vi "ATR.vi"() -> ()   [LabVIEW 2017]
panel:
  out "ATR 2":string[][](table)=[["Test Communication", "-", "-", "-", "-", ""], ["Set S/N", "-", "-", "-", "-", ""], ["Set Board Number", "-", "-", "-", "-", ""], [" ", "", "", "", "", ""], ["Test Communication", "-", "-", "-", "-", ""], ["Get S/N", "-", "-", "-", "", ""], ["Get Board Number", "-", "-", "-", "", ""], ["Get FW", "-", "-", "-", "", ""], ["Enable Motor", "", "", "", "", ""], ["Small position command", "", "", "", "", ""], ["Measure delta", "", "", "", "", ""], ["Velocity command", "", "", "", "", ""]] caption="ATR"
  out "ATR":string[][](table)=[["Test Communication", "-", "-", "-", "-", ""], ["Set S/N", "-", "-", "-", "-", ""], ["Set Board Number", "-", "-", "-", "-", ""], [" ", "", "", "", "", ""], ["Test Communication", "-", "-", "-", "-", ""], ["Get S/N", "-", "-", "-", "", ""], ["Get Board Number", "-", "-", "-", "", ""], ["Get FW", "-", "-", "-", "", ""], ["Enable Motor", "", "", "", "", ""], ["Small position command", "", "", "", "", ""], ["Measure delta", "", "", "", "", ""], ["Velocity command", "", "", "", "", ""]]
  out "Array 2":string[](array[string])
  out "Array":string[](array[string])
  out "deleted portion 2":string[](array[string])
  out "deleted portion":string[](array[string])
  out "ArrAHU":string[][](array[string])
  out "ArrEbay":string[][](array[string])
  out "Mort Temp":string[][](array[string])
  out "Aux":string[][](array[string])
  out "Burnin":string[][](array[string])
  out "Temp Algo":string[][](array[string])
  out "Speed":string[][](array[string])
  out "Tempreature calibration":string[][](array[string])
  out "StopTime":string[][](array[string])
  out "Enable":string[][](array[string])
  out "Communication":string[][](array[string])
  out "Visual Inspection":string[][](array[string])
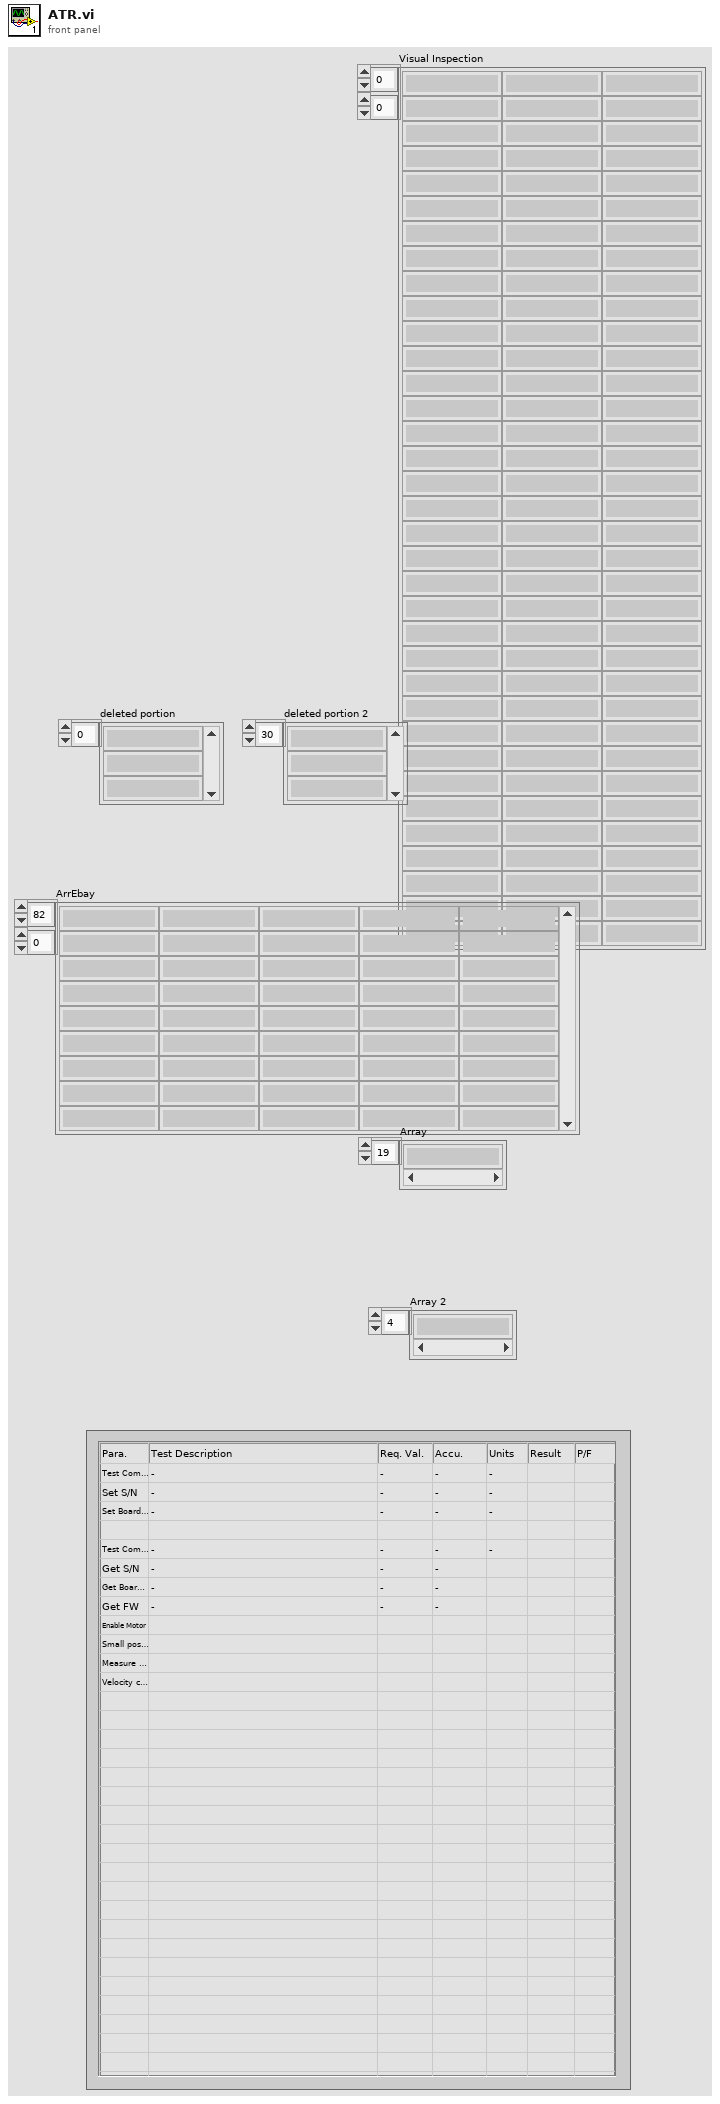
[diagram p1: front panel]
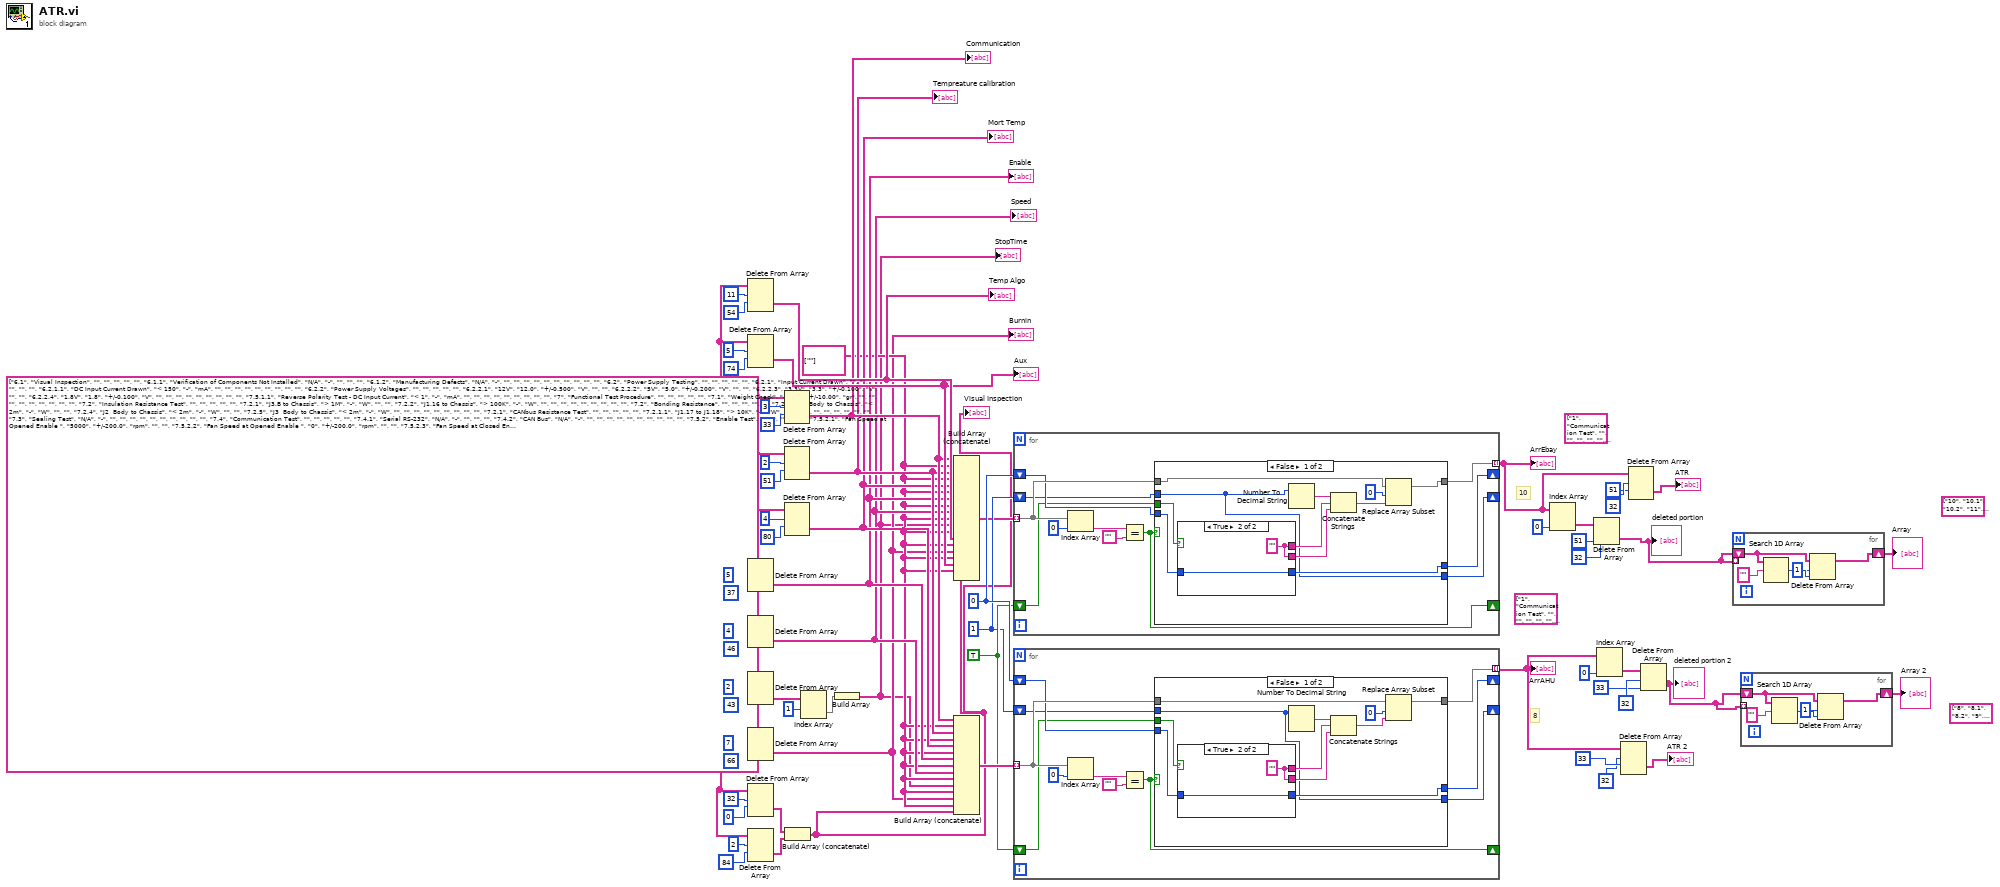
[diagram p0: block diagram]
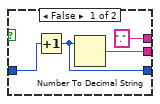
[diagram p2: hidden frame]
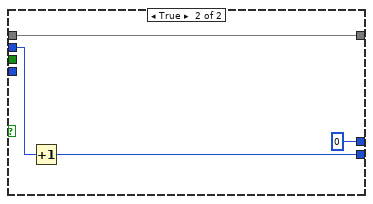
[diagram p3: hidden frame]
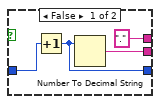
[diagram p4: hidden frame]
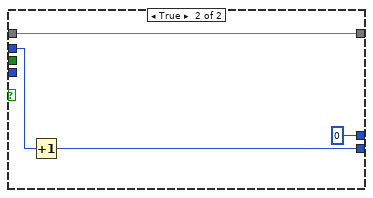
[diagram p5: hidden frame]
diagram:
  (unwired) string[] ["8", "8.1", "8.2", "9", "9.1", "9.2", "10", "10.1", "10.2", "10.3", "10.4", "11", "12", "12.1", "13", "13.1", "13.2", "14", "14.1", "14.2", "14.3", "15", "15.1", "16"] ("Array 3")
  (unwired) string[] ["10", "10.1", "10.2", "11", "11.1", "11.2", "12", "12.1", "12.2", "12.3", "12.4", "13", "14", "14.1", "15", "15.1", "15.2", "16", "16.1", "16.2", "16.3", "17", "17.1", "18"] ("Array 4")
  (unwired) string[][] [["1", "Communication Test", "", "", "", "", ""], ["1.1", "Serial RS-232", "N/A", "-", "", "", ""], ["1.2", "CAN Bus", "N/A", "-", "", "", ""], ["", "", "", "", "", "", ""], ["2", "Temperature Sensor Calibration", "", "", "", "", ""], ["2.1", "Sensor Reading Analog Offset", "0", "+/-0.100", ".", "", ""], ["", "", "", "", "", "", ""], ["3", "Motor Termistor Input Test", "", "", "", "", ""], ["3.1", "60 Degree", "60", "+/-3.00", "C", "", ""], ["3.2", "90 Degree", "90", "+/-3.00", "C", "", ""], ["3.3", "120 Degree", "120", "+/-3.00", "C", "", ""], ["", "", "", "", "", "", ""], ["4", "Enable Test", "", "", "", "", ""], ["4.1", "Fan Speed at Opened Enable ", "5000", "+/-200.0", "rpm", "", ""], ["4.2", "Fan Speed at Opened Enable ", "0", "+/-200.0", "rpm", "", ""], ["4.3", "Fan Speed at Closed Enable ", "5000", "+/-200.0", "rpm", "", ""], ["4.4", "Motor Rotation Direction", "Counter-clockwise (Inlet)", "-", "", "", ""], ["", "", "", "", "", "", ""], ["5", "Speed Command Test", "", "", "", "", ""], ["5.1", "Fan Speed", "6000", "+/-200.0", "rpm", "", ""], ["5.2", "Fan Speed", "11500", "+/-200.0", "rpm", "", ""], ["5.3", "Fan Speed", "15100", "+/-200.0", "rpm", "", ""], ["", "", "", "", "", "", ""], ["6", "Motor Stop time", "< 50", "-", "sec", "", ""], ["", "", "", "", "", "", ""], ["7", "Temperature Control Algorithm Test", "", "", "", "", ""], ["7.1", "Tair <   68 ± 2 oC", "6000", "+/-200.0", "rpm", "", ""], ["7.2", "Measured Temp.", "", "", "C", "", ""], ["7.3", "Tair >= 68 ± 2 oC", "11500", "+/-200.0", "rpm", "", ""], ["7.4", "Transition Temp.", "", "", "C", "", ""], ["7.5", "Tair >= 88 ± 2 oC", "15100", "+/-400.0", "rpm", "", ""], ["7.6", "Transition Temp.", "", "", "C", "", ""], ["7.7", "Tair <= 80 ± 2 oC", "11500", "+/-200.0", "rpm", "", ""], ["7.8", "Transition Temp.", "", "", "C", "", ""], ["7.9", "Tair <= 60 ± 2 oC", "6000", "+/-200.0", "rpm", "", ""], ["7.10", "Transition Temp.", "", "", "C", "", ""], ["", "", "", "", "", "", ""], ["8", "Burn-in Test", "", "", "", "", ""], ["8.1", "DC Input Current", "50", "+/-5.000", "A", "", ""], ["8.2", "Fan Speed", "15100", "+/-200.0", "rpm", "", ""], ["8.3", "Ambient Temperature", "25", "+/-13.00", "C", "", ""], ["8.4", "After 10 min of operation", "", "-", "C", "", ""], ["8.5", "After 20 min of operation", "", "-", "C", "", ""], ["8.6", "After 30 min of operation", "", "-", "C", "", ""], ["", "", "", "", "", "", ""], ["9", "Auxiliary Fan Test", "", "", "", "", ""], ["9.1", "Auxiliary Cooling Fan ON", "60", "+/-2.00", "C", "", ""], ["9.2", "Fan status", "ON", "-", "-", "", ""], ["9.3", "Auxiliary Cooling Fan OFF", "55", "+/-2.00", "C", "", ""], ["9.4", "Fan status", "OFF", "-", "-", "", ""], ["", "", "", "", "", "", ""], ["10", "Visual Inspection", "", "", "", "", ""], ["10.1", "Verification of Components Not Installed", "N/A", "-", "", "", ""], ["10.2", "Manufacturing Defects", "N/A", "-", "", "", ""], ["", "", "", "", "", "", ""], ["11", "Power Supply Testing", "", "", "", "", ""], ["11.1", "Input Current Drawn", "", "", "", "", ""], ["11.2", "DC Input Current", "< 150", "-", "mA", "", ""], ["", "", "", "", "", "", ""], ["12", "Power Supply Voltages", "", "", "", "", ""], ["12.1", "12V", "12.0", "+/-0.500", "V", "", ""], ["12.2", "5V", "5.0", "+/-0.200", "V", "", ""], ["12.3", "3.3V", "3.3", "+/-0.100", "V", "", ""], ["12.4", "1.8V", "1.8", "+/-0.100", "V", "", ""], ["", "", "", "", "", "", ""], ["13", "Reverse Polarity Test - DC Input Current", "< 1", "-", "mA", "", ""], ["", "", "", "", "", "", ""], ["14", "Functional Test Procedure", "", "", "", "", ""], ["14.1", "Weight Check", "4180", "+/-10.00", "gr", "", ""], ["", "", "", "", "", "", ""], ["15", "Insulation Resistance Test", "", "", "", "", ""], ["15.1", "J3.B to Chassis", "> 1M", "-", "W", "", ""], ["15.2", "J1.16 to Chassis", "> 100K", "-", "W", "", ""], ["", "", "", "", "", "", ""], ["16", "Bonding Resistance", "", "", "", "", ""], ["16.1", "J1 Body to Chassis", "< 2m", "-", "W", "", ""], ["16.2", "J2  Body to Chassis", "< 2m", "-", "W", "", ""], ["16.3", "J3  Body to Chassis", "< 2m", "-", "W", "", ""], ["", "", "", "", "", "", ""], ["17", "CANbus Resistance Test", "", "", "", "", ""], ["17.1", "J1.17 to J1.18", "> 10K", "-", "W", "", ""], ["", "", "", "", "", "", ""], ["18", "Sealing Test", "N/A", "-", "", "", ""]] ("ArrEbay 2")
  (unwired) string[][] [["1", "Communication Test", "", "", "", "", ""], ["1.1", "Serial RS-232", "N/A", "-", "", "", ""], ["1.2", "CAN Bus", "N/A", "-", "", "", ""], ["", "", "", "", "", "", ""], ["2", "Temperature Sensor Calibration", "", "", "", "", ""], ["2.1", "Sensor Reading Analog Offset", "0", "+/-0.100", ".", "", ""], ["", "", "", "", "", "", ""], ["3", "Motor Termistor Input Test", "", "", "", "", ""], ["3.1", "60 Degree", "60", "+/-3.00", "C", "", ""], ["3.2", "90 Degree", "90", "+/-3.00", "C", "", ""], ["3.3", "120 Degree", "120", "+/-3.00", "C", "", ""], ["", "", "", "", "", "", ""], ["4", "Enable Test", "", "", "", "", ""], ["4.1", "Fan Speed at Opened Enable ", "5000", "+/-200.0", "rpm", "", ""], ["4.2", "Fan Speed at Opened Enable ", "0", "+/-200.0", "rpm", "", ""], ["4.3", "Fan Speed at Closed Enable ", "5000", "+/-200.0", "rpm", "", ""], ["4.4", "Motor Rotation Direction", "Counter-clockwise (Inlet)", "-", "", "", ""], ["", "", "", "", "", "", ""], ["5", "Speed Command Test", "", "", "", "", ""], ["5.1", "Fan Speed", "6000", "+/-200.0", "rpm", "", ""], ["5.2", "Fan Speed", "11500", "+/-200.0", "rpm", "", ""], ["5.3", "Fan Speed", "15100", "+/-200.0", "rpm", "", ""], ["", "", "", "", "", "", ""], ["6", "Motor Stop time", "< 50", "-", "sec", "", ""], ["", "", "", "", "", "", ""], ["7", "Burn-in Test", "", "", "", "", ""], ["7.1", "DC Input Current", "50", "+/-5.000", "A", "", ""], ["7.2", "Fan Speed", "15100", "+/-200.0", "rpm", "", ""], ["7.3", "Ambient Temperature", "25", "+/-13.00", "C", "", ""], ["7.4", "After 10 min of operation", "", "-", "C", "", ""], ["7.5", "After 20 min of operation", "", "-", "C", "", ""], ["7.6", "After 30 min of operation", "", "-", "C", "", ""], ["", "", "", "", "", "", ""], ["8", "Visual Inspection", "", "", "", "", ""], ["8.1", "Verification of Components Not Installed", "N/A", "-", "", "", ""], ["8.2", "Manufacturing Defects", "N/A", "-", "", "", ""], ["", "", "", "", "", "", ""], ["9", "Power Supply Testing", "", "", "", "", ""], ["9.1", "Input Current Drawn", "", "", "", "", ""], ["9.2", "DC Input Current", "< 150", "-", "mA", "", ""], ["", "", "", "", "", "", ""], ["10", "Power Supply Voltages", "", "", "", "", ""], ["10.1", "12V", "12.0", "+/-0.500", "V", "", ""], ["10.2", "5V", "5.0", "+/-0.200", "V", "", ""], ["10.3", "3.3V", "3.3", "+/-0.100", "V", "", ""], ["10.4", "1.8V", "1.8", "+/-0.100", "V", "", ""], ["", "", "", "", "", "", ""], ["11", "Reverse Polarity Test - DC Input Current", "< 1", "-", "mA", "", ""], ["", "", "", "", "", "", ""], ["12", "Functional Test Procedure", "", "", "", "", ""], ["12.1", "Weight Check", "4180", "+/-10.00", "gr", "", ""], ["", "", "", "", "", "", ""], ["13", "Insulation Resistance Test", "", "", "", "", ""], ["13.1", "J3.B to Chassis", "> 1M", "-", "W", "", ""], ["13.2", "J1.16 to Chassis", "> 100K", "-", "W", "", ""], ["", "", "", "", "", "", ""], ["14", "Bonding Resistance", "", "", "", "", ""], ["14.1", "J1 Body to Chassis", "< 2m", "-", "W", "", ""], ["14.2", "J2  Body to Chassis", "< 2m", "-", "W", "", ""], ["14.3", "J3  Body to Chassis", "< 2m", "-", "W", "", ""], ["", "", "", "", "", "", ""], ["15", "CANbus Resistance Test", "", "", "", "", ""], ["15.1", "J1.17 to J1.18", "> 10K", "-", "W", "", ""], ["", "", "", "", "", "", ""], ["16", "Sealing Test", "N/A", "-", "", "", ""]] ("ArrAHU 2")
  w37 = string[][] [[""]] ("array")
  w34 = TRUE
  w33 = 1
  w35 = 0
  w4 = string[][] [["6.1", "Visual Inspection", "", "", "", "", ""], ["6.1.1", "Verification of Components Not Installed", "N/A", "-", "", "", ""], ["6.1.2", "Manufacturing Defects", "N/A", "-", "", "", ""], ["", "", "", "", "", "", ""], ["6.2", "Power Supply Testing", "", "", "", "", ""], ["6.2.1", "Input Current Drawn", "", "", "", "", ""], ["6.2.1.1", "DC Input Current Drawn", "< 150", "-", "mA", "", ""], ["", "", "", "", "", "", ""], ["6.2.2", "Power Supply Voltages", "", "", "", "", ""], ["6.2.2.1", "12V", "12.0", "+/-0.500", "V", "", ""], ["6.2.2.2", "5V", "5.0", "+/-0.200", "V", "", ""], ["6.2.2.3", "3.3V", "3.3", "+/-0.100", "V", "", ""], ["6.2.2.4", "1.8V", "1.8", "+/-0.100", "V", "", ""], ["", "", "", "", "", "", ""], ["7.5.1.1", "Reverse Polarity Test - DC Input Current", "< 1", "-", "mA", "", ""], ["", "", "", "", "", "", ""], ["7", "Functional Test Procedure", "", "", "", "", ""], ["7.1", "Weight Check", "4180", "+/-10.00", "gr", "", ""], ["", "", "", "", "", "", ""], ["7.2", "Insulation Resistance Test", "", "", "", "", ""], ["7.2.1", "J3.B to Chassis", "> 1M", "-", "W", "", ""], ["7.2.2", "J1.16 to Chassis", "> 100K", "-", "W", "", ""], ["", "", "", "", "", "", ""], ["7.2", "Bonding Resistance", "", "", "", "", ""], ["7.2.3", "J1 Body to Chassis", "< 2m", "-", "W", "", ""], ["7.2.4", "J2  Body to Chassis", "< 2m", "-", "W", "", ""], ["7.2.5", "J3  Body to Chassis", "< 2m", "-", "W", "", ""], ["", "", "", "", "", "", ""], ["7.2.1", "CANbus Resistance Test", "", "", "", "", ""], ["7.2.1.1", "J1.17 to J1.18", "> 10K", "-", "W", "", ""], ["", "", "", "", "", "", ""], ["7.3", "Sealing Test", "N/A", "-", "", "", ""], ["", "", "", "", "", "", ""], ["7.4", "Communication Test", "", "", "", "", ""], ["7.4.1", "Serial RS-232", "N/A", "-", "", "", ""], ["7.4.2", "CAN Bus", "N/A", "-", "", "", ""], ["", "", "", "", "", "", ""], ["7.5.2", "Enable Test", "", "", "", "", ""], ["7.5.2.1", "Fan Speed at Opened Enable ", "5000", "+/-200.0", "rpm", "", ""], ["7.5.2.2", "Fan Speed at Opened Enable ", "0", "+/-200.0", "rpm", "", ""], ["7.5.2.3", "Fan Speed at Closed Enable ", "5000", "+/-200.0", "rpm", "", ""], ["7.5.2.4", "Motor Rotation Direction", "Counter-clockwise (Inlet)", "-", "", "", ""], ["", "", "", "", "", "", ""], ["7.5.3", "Stop Time Test ", "", "", "", "", ""], ["7.5.3.1", "Motor Stop time", "< 50", "-", "sec", "", ""], ["", "", "", "", "", "", ""], ["7.5.4", "Speed Command Test", "", "", "", "", ""], ["7.5.4.1", "Fan Speed", "6000", "+/-200.0", "rpm", "", ""], ["7.5.4.2", "Fan Speed", "11500", "+/-200.0", "rpm", "", ""], ["7.5.4.3", "Fan Speed", "15100", "+/-200.0", "rpm", "", ""], ["", "", "", "", "", "", ""], ["7.5.5", "Temperature Sensor Calibration", "", "", "", "", ""], ["7.5.5.1", "Sensor Reading Analog Offset", "0", "+/-0.100", ".", "", ""], ["", "", "", "", "", "", ""], ["7.5.6", "Temperature Control Algorithm Test", "", "", "", "", ""], ["7.5.6.1", "Tair <   68 ± 2 oC", "6000", "+/-200.0", "rpm", "", ""], ["7.5.6.2", "Measured Temp.", "", "", "C", "", ""], ["7.5.6.3", "Tair >= 68 ± 2 oC", "11500", "+/-200.0", "rpm", "", ""], ["7.5.6.4", "Transition Temp.", "", "", "C", "", ""], ["7.5.6.5", "Tair >= 88 ± 2 oC", "15100", "+/-400.0", "rpm", "", ""], ["7.5.6.6", "Transition Temp.", "", "", "C", "", ""], ["7.5.6.7", "Tair <= 80 ± 2 oC", "11500", "+/-200.0", "rpm", "", ""], ["7.5.6.8", "Transition Temp.", "", "", "C", "", ""], ["7.5.6.9", "Tair <= 60 ± 2 oC", "6000", "+/-200.0", "rpm", "", ""], ["7.5.6.10", "Transition Temp.", "", "", "C", "", ""], ["", "", "", "", "", "", ""], ["7.5.7", "Burn-in Test", "", "", "", "", ""], ["7.5.7.1", "DC Input Current", "50", "+/-5.000", "A", "", ""], ["7.5.7.2", "Fan Speed", "15100", "+/-200.0", "rpm", "", ""], ["7.5.7.3", "Ambient Temperature", "25", "+/-13.00", "C", "", ""], ["7.5.7.4", "After 10 min of operation", "", "-", "C", "", ""], ["7.5.7.5", "After 20 min of operation", "", "-", "C", "", ""], ["7.5.7.6", "After 30 min of operation", "", "-", "C", "", ""], ["", "", "", "", "", "", ""], ["8", "Auxiliary Fan Test", "", "", "", "", ""], ["8.1", "Auxiliary Cooling Fan ON", "60", "+/-2.00", "C", "", ""], ["8.2", "Fan status", "ON", "-", "-", "", ""], ["8.3", "Auxiliary Cooling Fan OFF", "55", "+/-2.00", "C", "", ""], ["8.4", "Fan status", "OFF", "-", "-", "", ""], ["", "", "", "", "", "", ""], ["9", "Motor Termistor Input Test", "", "", "", "", ""], ["9.1", "60 Degree", "60", "+/-3.00", "C", "", ""], ["9.2", "90 Degree", "90", "+/-3.00", "C", "", ""], ["9.3", "120 Degree", "120", "+/-3.00", "C", "", ""], ["", "", "", "", "", "", ""], ["10", "Mounting Holes Test - Jig Fit", "214", "-", "mm", "", ""]] ("data")
  # "8"
  # "10"
  n1 = Delete From Array(array=w4, length=11, index (row)=54) -> (deleted portion=w44:string[][])  [unwired: 1 in, 1 out]
  "Temp Algo" <- w44
  n2 = Delete From Array(array=w4, length=5, index (row)=74) -> (deleted portion=w43:string[][])  [unwired: 1 in, 1 out]
  "Aux" <- w43
  n3 = Delete From Array(array=w4, length=5, index (row)=37) -> (deleted portion=w39:string[][])  [unwired: 1 in, 1 out]
  "Enable" <- w39
  n4 = Delete From Array(array=w4, length=4, index (row)=46) -> (deleted portion=w38:string[][])  [unwired: 1 in, 1 out]
  "Speed" <- w38
  n5 = Delete From Array(array=w4, length=2, index (row)=43) -> (deleted portion=w30:string[][])  [unwired: 1 in, 1 out]
  n6 = Delete From Array(array=w4, length=7, index (row)=66) -> (deleted portion=w31:string[][])  [unwired: 1 in, 1 out]
  "Burnin" <- w31
  n7 = Delete From Array(array=w4, length=32, index (row)=0) -> (deleted portion=w3:string[][])  [unwired: 1 in, 1 out]
  n8 = Delete From Array(array=w4, length=2, index (row)=84) -> (deleted portion=w2:string[][])  [unwired: 1 in, 1 out]
  n9 = Delete From Array(array=w4, length=3, index (row)=33) -> (deleted portion=w42:string[][])  [unwired: 1 in, 1 out]
  "Communication" <- w42
  n10 = Delete From Array(array=w4, length=2, index (row)=51) -> (deleted portion=w41:string[][])  [unwired: 1 in, 1 out]
  "Tempreature calibration" <- w41
  n11 = Delete From Array(array=w4, length=4, index (row)=80) -> (deleted portion=w40:string[][])  [unwired: 1 in, 1 out]
  "Mort Temp" <- w40
  n12 = Build Array (concatenate)(w3, w2) -> (w1:string[][])
  "Visual Inspection" <- w1
  n13 = Index Array(array=w30, index (row)=1) -> (element=w28:string[])  [unwired: 1 in]
  n14 = Build Array(w28) -> (w27:string[][])
  "StopTime" <- w27
  n15 = Build Array (concatenate)(w42, w37, w41, w37, w40, w37, w39, w37, w38, w37, w27, w37, w44, w37, w31, w37, w43, w37, w1) -> (w32:string[][])
  n16 = Build Array (concatenate)(w42, w37, w41, w37, w40, w37, w39, w37, w38, w37, w27, w37, w31, w37, w1) -> (w36:string[][])
  n17 = for {
    tunnel: w32 -> [w74] mode=indexing
    tunnel: [w75] -> w12 mode=indexing
    shift-right: [w69] -> _
    shift-left: w35 -> [w70]
    shift-right: [w67] -> _
    shift-left: w33 -> [w68]
    shift-right: [w66] -> _
    shift-left: w34 -> [w65]
    n18 = Index Array(array=w74, index=0) -> (element=w72:string)
    n19 = Equal?(x=w72, y="") -> (x = y?=w66:bool)
    n20 = case shown="False" w66 {
      tunnel: w70 -> [w80 _]
      tunnel: [w83 w96] -> w75
      tunnel: w74 -> [w82 w96]
      tunnel: [w81 0] -> w69
      tunnel: w68 -> [w77 w95]
      tunnel: [w77 w94] -> w67
      tunnel: w65 -> [w76 _]
      frame False {
        n21 = case shown="True" w76 {
          tunnel: [w90 w92] -> w85
          tunnel: [w89 w91] -> w81
          tunnel: w80 -> [w88 w91]
          tunnel: ["." ("string") w92] -> w78
          frame False {
            n22 = Increment(x=w88) -> (x+1=w89:i32)
            n23 = Number To Decimal String(number=w89) -> (decimal integer string=w90:string)  [unwired: 1 in]
          }
          frame True {
            w92 = "" ("string")
          }
        }
        n24 = Number To Decimal String(number=w77) -> (decimal integer string=w79:string)  [unwired: 1 in]
        n25 = Concatenate Strings(w79, w78, w85) -> (w84:string)
        n26 = Replace Array Subset(array=w82, new element=w84, index=0) -> (w83:string[])
      }
      frame True {
        n27 = Increment(x=w95) -> (x+1=w94:i32)
      }
    }
  }
  "ArrEbay" <- w12
  n28 = for {
    tunnel: w36 -> [w106] mode=indexing
    tunnel: [w107] -> w7 mode=indexing
    shift-right: [w101] -> _
    shift-left: w35 -> [w102]
    shift-right: [w99] -> _
    shift-left: w33 -> [w100]
    shift-right: [w98] -> _
    shift-left: w34 -> [w97]
    n29 = Index Array(array=w106, index=0) -> (element=w104:string)
    n30 = Equal?(x=w104, y="") -> (x = y?=w98:bool)
    n31 = case shown="False" w98 {
      tunnel: w102 -> [w112 _]
      tunnel: [w115 w128] -> w107
      tunnel: w106 -> [w114 w128]
      tunnel: [w113 0] -> w101
      tunnel: w100 -> [w109 w127]
      tunnel: [w109 w126] -> w99
      tunnel: w97 -> [w108 _]
      frame False {
        n32 = case shown="True" w108 {
          tunnel: [w122 w124] -> w117
          tunnel: [w121 w123] -> w113
          tunnel: w112 -> [w120 w123]
          tunnel: ["." ("string") w124] -> w110
          frame False {
            n33 = Increment(x=w120) -> (x+1=w121:i32)
            n34 = Number To Decimal String(number=w121) -> (decimal integer string=w122:string)  [unwired: 1 in]
          }
          frame True {
            w124 = "" ("string")
          }
        }
        n35 = Number To Decimal String(number=w109) -> (decimal integer string=w111:string)  [unwired: 1 in]
        n36 = Concatenate Strings(w111, w110, w117) -> (w116:string)
        n37 = Replace Array Subset(array=w114, new element=w116, index=0) -> (w115:string[])
      }
      frame True {
        n38 = Increment(x=w127) -> (x+1=w126:i32)
      }
    }
  }
  "ArrAHU" <- w7
  n39 = Index Array(array=w12, index (col)=0 ("disabled index (col)")) -> (element=w25:string[])  [unwired: 1 in]
  n40 = Delete From Array(array=w25, length=32, index=51) -> (deleted portion=w18:string[])  [unwired: 1 out]
  "deleted portion" <- w18
  n41 = Index Array(array=w7, index (col)=0 ("disabled index (col)")) -> (element=w20:string[])  [unwired: 1 in]
  n42 = Delete From Array(array=w7, length=32, index (row)=33 ("index")) -> (deleted portion=→"ATR 2":string[][])  [unwired: 1 in, 1 out]
  n43 = Delete From Array(array=w12, length=32, index (row)=51 ("index")) -> (deleted portion=→"ATR":string[][])  [unwired: 1 in, 1 out]
  n44 = Delete From Array(array=w20, length=32, index=33) -> (deleted portion=w15:string[])  [unwired: 1 out]
  "deleted portion 2" <- w15
  n45 = for {
    tunnel: w18 -> [_] mode=indexing
    shift-right: [w129] -> w17
    shift-left: w18 -> [w132]
    n46 = Search 1D Array(1D array=w132, element="") -> (index of element=w131:i32)  [unwired: 1 in]
    n47 = Delete From Array(array=w132, length=1, index=w131) -> (array with subset deleted=w129:string[])  [unwired: 1 out]
  }
  "Array" <- w17
  n48 = for {
    shift-right: [w134] -> w16
    shift-left: w15 -> [w137]
    tunnel: w15 -> [_] mode=indexing
    n49 = Search 1D Array(1D array=w137, element="") -> (index of element=w136:i32)  [unwired: 1 in]
    n50 = Delete From Array(array=w137, length=1, index=w136) -> (array with subset deleted=w134:string[])  [unwired: 1 out]
  }
  "Array 2" <- w16
